vi "Write B scans.vi"(8 "error in (no error)":errorcluster, 10 "B scans":dbl=300.0, 11 "Scan in":refnum<class "Scan.lvclass">) -> (0 "error out":errorcluster, 3 "Scan out":refnum<class "Scan.lvclass">)   [LabVIEW 2017, in "Scan.lvclass"]
uses:
  Scan.lvclass
  Scan.lvclass/Scan.ctl
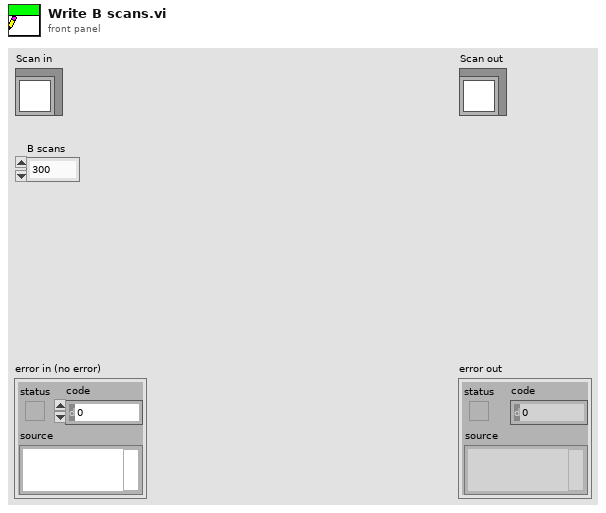
[diagram p1: front panel]
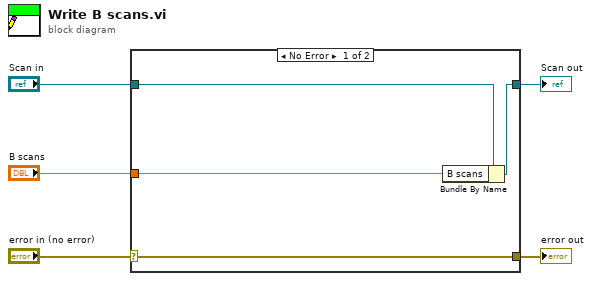
[diagram p0: block diagram]
diagram:
  n1 = case shown="No Error" "error in (no error)" {
    selector: "error in (no error)" -> [w9 w10]
    tunnel: [w9 w10] -> w4
    tunnel: [w7 w11] -> w2
    tunnel: "Scan in" -> [w8 w11]
    tunnel: "B scans" -> [w6 _]
    frame No Error {
      n2 = Bundle By Name(cluster=w8, "B scans"=w6) -> (w7:refnum<class "Scan.lvclass">)
    }
    frame Error {
    }
  }
  "error out" <- w4
  "Scan out" <- w2
